vi "PH_SSAC.panel.vi"(0 "object ref":refnum<vi>, 5 "error in (no error)":errorcluster) -> (19 "error out":errorcluster)   [LabVIEW 2014, in "PH_SSAC.lvlib"]
doc: "This a GUI.\n\nLicense Agreement for this software:\n\nCopyright (C)\nGesellschaft für Schwerionenforschung, GSI\nPlanckstr. 1\n64291 Darmstadt\nGermany\n\nContact: D.Beck@gsi.de \n\nThis program is free software; you can redistribute it and/or modify it under the terms of the GNU General Public License as published by the Free Software Foundation; either version 2 of the license, or (at your option) any later version.\n\nThis program is distributed in the hope that it will be useful, but WITHOUT ANYW ARRANTY; without even the implied warranty of MERCHANTABILITY or FITNESS FOR A PARTICULAR PURPOSE. See the GNU General License for more details (http://www.gnu.org).\n\nGesellschaft für Schwerionenforschung, GSI\nPlanckstr. 1, 64291 Darmstadt, Germany\nFor all questions and ideas contact: M.Richter@gsi.de, H.Brand@gsi.de or D.Beck@gsi.de.\nLast update: 18-DEC-2002"
uses:
  PH_SSAC.lvlib
  PH_Basics/PH_StatusHandler/PH_StatusHandler.GUI element.ctl
  PH_SSAC.Background Data.ctl
  PH_Basics/PH_Img_BaseClass/PH_Img_BaseClass.Palette.ctl
  PH_Basics/PH_Img_BaseClass/PH_Img_BaseClass.GUI Refs.ctl
  PH_SSAC.Signal Selector.ctl
  PH_Basics/PH_StatusHandler/PH_StatusHandler.Status.ctl
  CS_Core/CSObj/CSObj.lvlib
  PH_Basics/PH_Common/PH_Common.lvlib
  CS_Core/CSSystem/CSSystemLib/CSSystemLib.lvlib
  PH_Basics/PH_Img_BaseClass/PH_Img_BaseClass.lvlib
  PH_Basics/PH_Class/PH_Class.lvlib
  PH_Basics/PH_PSDBWriter/PH_PSDBWriter.lvlib
  PH_Basics/PH_StatusHandler/PH_StatusHandler.lvlib
panel:
  out "Background":u32(colorbox)=16860
  out "Timeout":u32(colorbox)=16860
  in  "Tab Control":T1(tab)=enum."Calibration"
  in  "Export Evaluation":bool caption="Export\nEvaluation"
  in  "# for Average":i32=1
  out "Saturation":bool
  out "Processed":bool
  in  "Threshold":dbl
  out "Mean Pulse Duration":dbl caption="fs"
  out "Current Pulse Duration":dbl caption="fs"
  out "Time evolution of mean pulse duration":dbl[](graph)
  out "Main signal":cluster{dbl[], "Main Signal":dbl[]}(graph)
  out "Calibration Factor":dbl caption="fs/pixel"
  in  "dt":dbl=1.0 caption="fs"
  out "Cam Source":string
  in  "Timeout Set":i32 caption="ms"
  in  "Global On":bool caption="On"
  in  "Palette":T2 items=["Grey", "Binary", "Gradient", "Rainbow", "Temperature"]
  out "GUI Image":T3(plugin-control)
  in  "Frame Main":cluster{"x":u32, "dx":u32, "y":u32, "dy":u32}={"x"=0, "dx"=1280, "y"=150, "dy"=150} caption="Main Signal"
  in  "Frame Background":cluster{"x":u32, "dx":u32, "y":u32, "dy":u32}={"x"=0, "dx"=100, "y"=400, "dy"=250} caption="Background"
  in  "Calibration Procedure":bool
  out "Background Calibration Data":T4={"Date"="", "Time"="", "Frame Main"={"x"=0, "dx"=0, "y"=0, "dy"=0}, "dt [fs]"=0.0, "Calibration Factor [fs/pixel]"=0.0, "Signal"=array[1280 elements], "Frame Background"={"x"=0, "dx"=100, "y"=400, "dy"=250}}
  in  "Read BG Data":bool
  in  "Save BG Data":bool
  out "Current Position":i32 caption="pixel"
  in  "Background acquire":bool
  out "Resulting Factor":dbl caption="fs/pixel"
  in  "Stage Pos 1":dbl caption="mm"
  in  "1st peak at":dbl caption="pixel"
  in  "2nd peak at":dbl caption="pixel"
  in  "Stage Pos 2":dbl caption="mm"
  in  "Calculate Factor":bool
  in  "Calibration Procedure Step":u16(ring)
  out "PSDB Status":u32(colorbox)=6618880 caption="PSDB"
  out "Status":T5 caption="Enabling State"
  in  "Delete":bool
  in  "Exit":bool
  # "PCS"
  # "3.40"
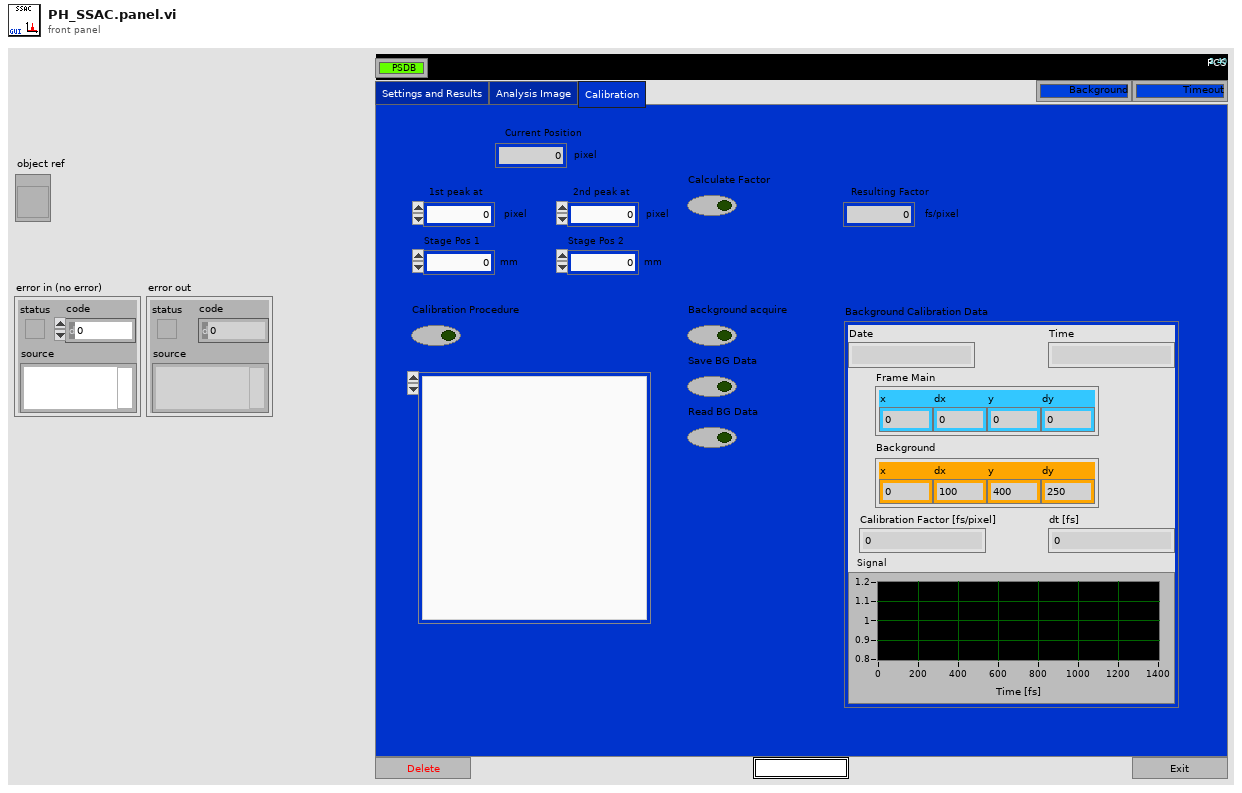
[diagram p1: front panel]
types:
  T1 = enum32{"Settings and Results", "Analysis Image", "Calibration"}
  T2 = typedef "PH_Img_BaseClass.lvlib/PH_Img_BaseClass.Palette.ctl" = i32
  T3 = typedef "IMAQ Image.ctl" = refnum<image>
  T4 = typedef "PH_SSAC.lvlib/PH_SSAC.Background Data.ctl" = cluster{"Date":string, "Time":string, "Frame Main":cluster{"x":u32, "dx":u32, "y":u32, "dy":u32}, "dt [fs]":dbl, "Calibration Factor [fs/pixel]":dbl, "Signal":dbl[], "Frame Background":cluster{"x":u32, "dx":u32, "y":u32, "dy":u32}}
  T5 = typedef "PH_StatusHandler.lvlib/PH_StatusHandler.GUI element.ctl" = u16
  T6 = typedef "PH_Img_BaseClass.lvlib/PH_Img_BaseClass.GUI Refs.ctl" = cluster{"Timeout":refnum<vi>, "Image":refnum<vi>, "Palette":refnum<vi>, "Timeout Set":refnum<vi>}
  T7 = typedef "PH_SSAC.lvlib/PH_SSAC.Signal Selector.ctl" = enum16{"Main", "Background"}
  T8 = typedef "PH_SSAC.lvlib/PH_SSAC.i attribute.ctl" = cluster{"GUI Refs":cluster{"Delete":refnum<vi>, "Global On":refnum<vi>, "Cam Source":refnum<vi>, "Frame Main Signal":refnum<vi>, "Frame Background":refnum<vi>, "dt (Gauss smooth)":refnum<vi>, "Calibration Factor":refnum<vi>, "Background acquire":refnum<vi>, "Threshold":refnum<vi>, "Time evolution of mean pulse duration":refnum<vi>, "Mean Pulse Duration":refnum<vi>, "Main signal":refnum<vi>, "Current Pulse Duration":refnum<vi>, "Processed":refnum<vi>, "Saturation":refnum<vi>, "# for Average":refnum<vi>, "Position":refnum<vi>, "BG Status":refnum<vi>, "Save BG data":refnum<vi>, "Read BG Data":refnum<vi>, "Background Calibration Data":refnum<vi>}, "Images":cluster{"OP Image":T3, "GUI Image":T3, "PSDB Image":T3}, "Global On?":bool, "Frame Main":cluster{"x":u32, "dx":u32, "y":u32, "dy":u32}, "Frame Background":cluster{"x":u32, "dx":u32, "y":u32, "dy":u32}, "dt [fs]":dbl, "Calibration Factor [fs/pixel]":dbl, "Threshold":dbl, "Time evolution of mean pulse duration [fs]":dbl[], "Main Signal":cluster{"Time for Main":dbl[], "Signal":dbl[]}, "Processed":bool, "Current Pulse Duration [fs]":dbl, "# for Average":i32, "Position":i32, "Pulse Durations [fs]":dbl[], "BG":cluster{"Acquire?":bool, "Background Calibration Data":T4, "Save Data":bool}}
  T9 = typedef "PH_StatusHandler.lvlib/PH_StatusHandler.Status.ctl" = i16
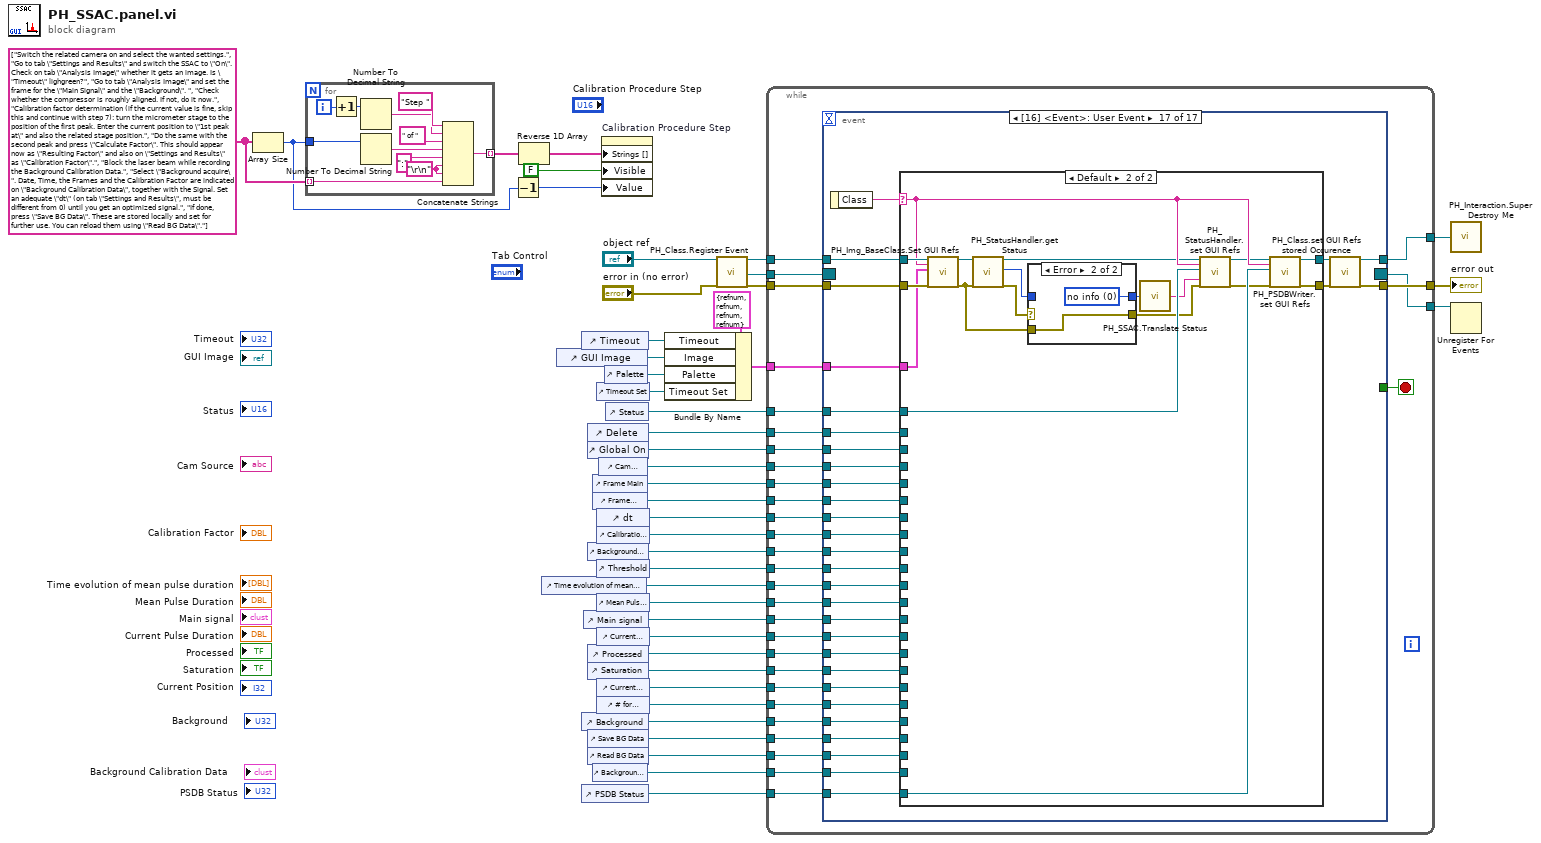
[diagram p0: block diagram]
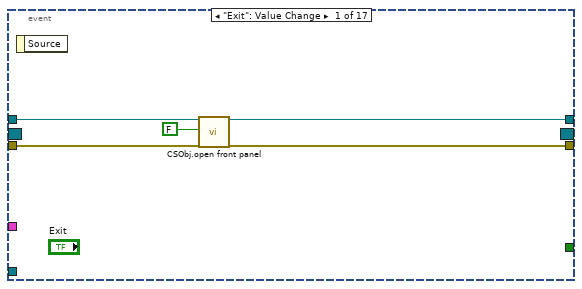
[diagram p2: hidden frame]
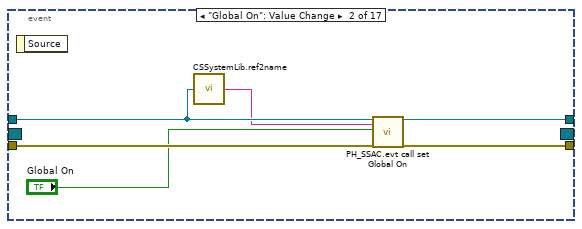
[diagram p3: hidden frame]
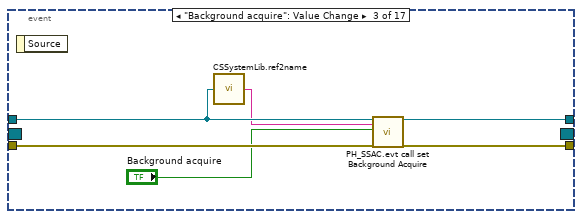
[diagram p4: hidden frame]
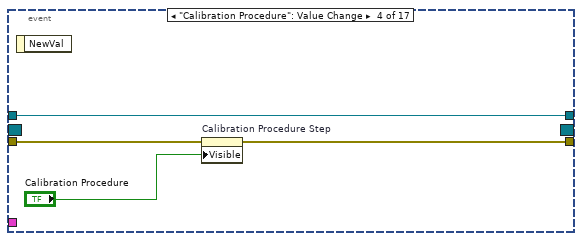
[diagram p5: hidden frame]
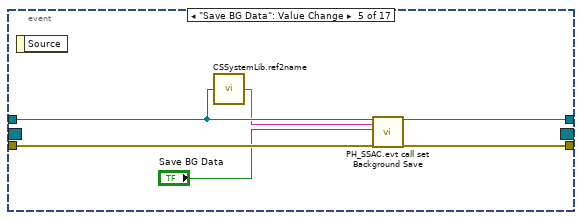
[diagram p6: hidden frame]
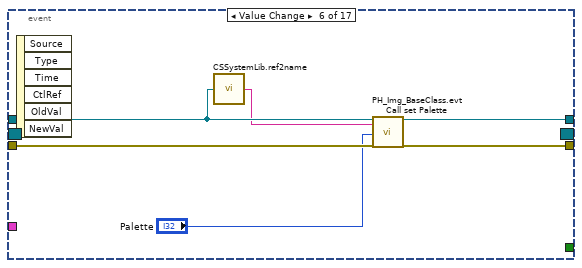
[diagram p7: hidden frame]
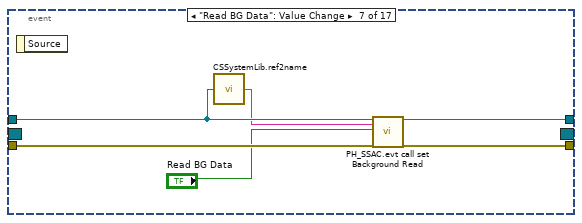
[diagram p8: hidden frame]
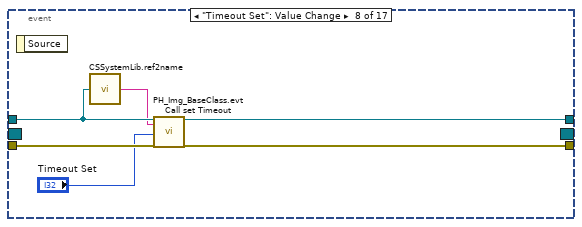
[diagram p9: hidden frame]
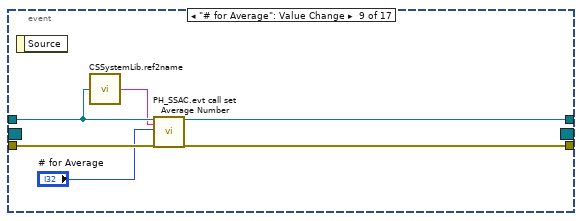
[diagram p10: hidden frame]
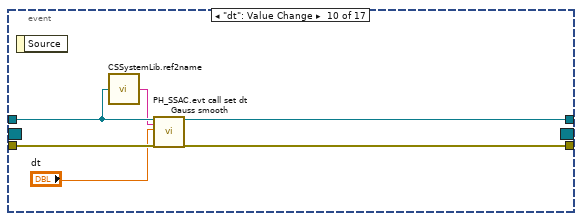
[diagram p11: hidden frame]
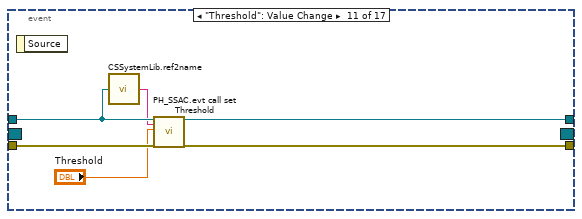
[diagram p12: hidden frame]
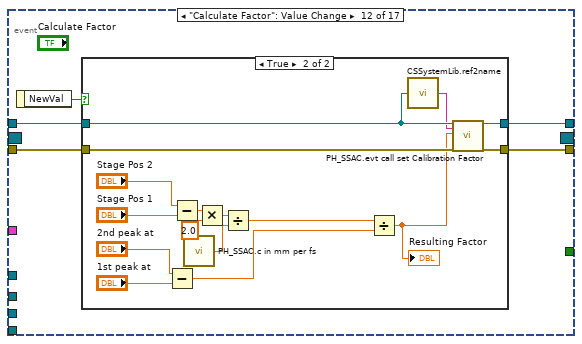
[diagram p13: hidden frame]
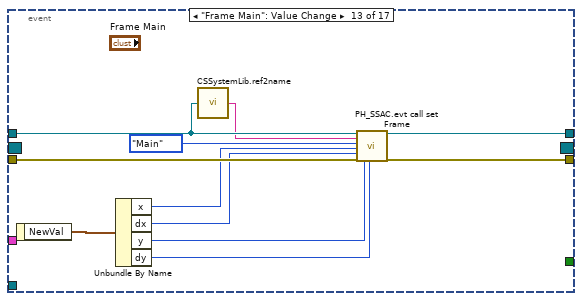
[diagram p15: hidden frame]
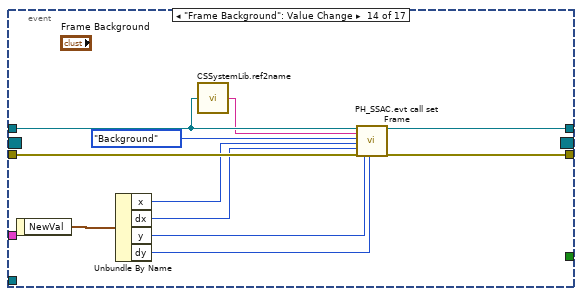
[diagram p16: hidden frame]
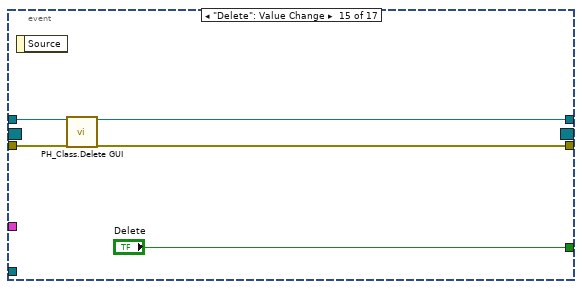
[diagram p17: hidden frame]
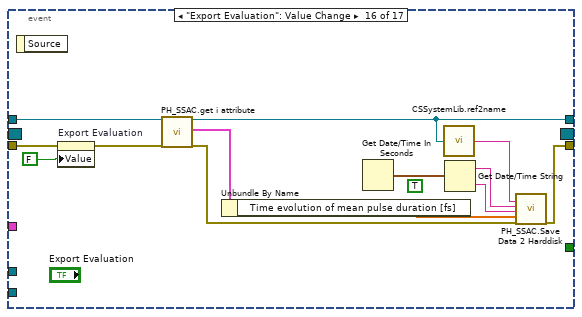
[diagram p18: hidden frame]
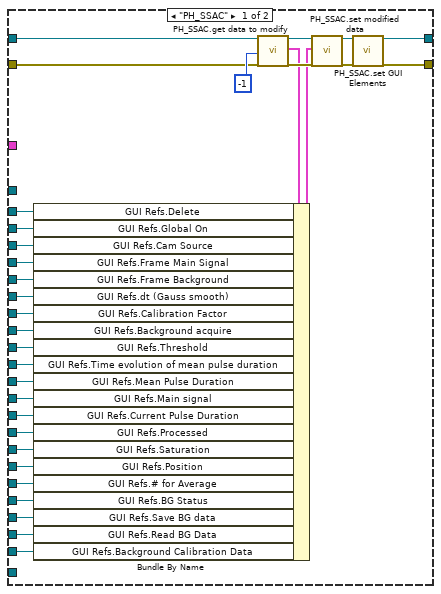
[diagram p19: hidden frame]
diagram:
  w40 = string[] ["Switch the related camera on and select the wanted settings.", "Go to tab \"Settings and Results\" and switch the SSAC to \"On\". Check on tab \"Analysis Image\" whether it gets an image. Is \"Timeout\" lighgreen?", "Go to tab \"Analysis Image\" and set the frame for the \"Main Signal\" and the \"Background\". ", "Check whether the compressor is roughly aligned. If not, do it now.", "Calibration factor determination (if the current value is fine, skip this and continue with step 7): turn the micrometer stage to the position of the first peak. Enter the current position to \"1st peak at\" and also the related stage position.", "Do the same with the second peak and press \"Calculate Factor\". This should appear now as \"Resulting Factor\" and also on \"Settings and Results\" as \"Calibration Factor\".", "Block the laser beam while recording the Background Calibration Data.", "Select \"Background acquire\". Date, Time, the Frames and the Calibration Factor are indicated on \"Background Calibration Data\", together with the Signal. Set an adequate \"dt\" (on tab \"Settings and Results\", must be different from 0) until you get an optimized signal.", "If done, press \"Save BG Data\". These are stored locally and set for further use. You can reload them using \"Read BG Data\"."]
  n1 = Array Size(array=w40) -> (size(s)=w36:i32)
  n2 = for {
    tunnel: w40 -> [w44] mode=indexing
    tunnel: [w53] -> w38 mode=indexing
    tunnel: w36 -> [w48]
    i -> [w52]
    w45 = "\r\n"
    n3 = Increment(x=w52) -> (x+1=w51:i32)
    n4 = Number To Decimal String(number=w51) -> (decimal integer string=w50:string)  [unwired: 1 in]
    n5 = Number To Decimal String(number=w48) -> (decimal integer string=w47:string)  [unwired: 1 in]
    n6 = Concatenate Strings("Step " ("string"), w50, " of " ("string"), w47, ":" ("string"), w45, w45, w44) -> (w53:string)
  }
  n7 = Decrement(x=w36) -> (x-1=w37:i32)
  n8 = Reverse 1D Array(array=w38) -> (reversed array=w39:string[])
  n9 = control-ref of="Time evolution of mean pulse duration"() -> (w16:refnum<vi>)
  n10 = control-ref of="GUI Image"() -> (w33:refnum<vi>)
  n11 = control-ref of="Timeout"() -> (w34:refnum<vi>)
  n12 = control-ref of="Background"() -> (w8:refnum<vi>)
  n13 = control-ref of="PSDB Status"() -> (w26:refnum<vi>)
  n14 = control-ref of="Main signal"() -> (w14:refnum<vi>)
  n15 = control-ref of="Delete"() -> (w25:refnum<vi>)
  n16 = control-ref of="Global On"() -> (w24:refnum<vi>)
  n17 = control-ref of="Background acquire"() -> (w18:refnum<vi>)
  n18 = control-ref of="Processed"() -> (w12:refnum<vi>)
  n19 = control-ref of="Saturation"() -> (w11:refnum<vi>)
  n20 = control-ref of="Save BG Data"() -> (w7:refnum<vi>)
  n21 = control-ref of="Read BG Data"() -> (w6:refnum<vi>)
  n22 = control-ref of="Frame Main"() -> (w22:refnum<vi>)
  n23 = control-ref of="Frame Background"() -> (w21:refnum<vi>)
  n24 = control-ref of="Background Calibration Data"() -> (w5:refnum<vi>)
  n25 = control-ref of="Timeout Set"() -> (w31:refnum<vi>)
  n26 = control-ref of="dt"() -> (w20:refnum<vi>)
  n27 = control-ref of="Calibration Factor"() -> (w19:refnum<vi>)
  n28 = control-ref of="Threshold"() -> (w17:refnum<vi>)
  n29 = control-ref of="Mean Pulse Duration"() -> (w15:refnum<vi>)
  n30 = control-ref of="Current Pulse Duration"() -> (w13:refnum<vi>)
  n31 = control-ref of="Current Position"() -> (w10:refnum<vi>)
  n32 = control-ref of="# for Average"() -> (w9:refnum<vi>)
  n33 = control-ref of="Cam Source"() -> (w23:refnum<vi>)
  n34 = property on="Calibration Procedure Step" class="Ring (strict)"("Strings []"=w39, "Visible"=FALSE, "Value"=w37) -> ()  [unwired: 2 in, 2 out]
  n35 = control-ref of="Palette"() -> (w32:refnum<vi>)
  n36 = control-ref of="Status"() -> (w1:refnum<vi>)
  n37 = Bundle By Name(cluster=T6 {"Timeout"=refnum, "Image"=refnum, "Palette"=refnum, "Timeout Set"=refnum} ("GUI Refs"), "Timeout"=w34, "Image"=w33, "Palette"=w32, "Timeout Set"=w31) -> (w4:T6)
  n38 = call "PH_Class.Register Event.vi"("i ref in"="object ref", "error in (no error)"="error in (no error)") -> ("i ref out"=w29:refnum<vi>, "Event Registration Refnum"=w28:refnum<event-registration>, "error out"=w30:errorcluster)  [unwired: 15 in]
  n39 = while {
    tunnel: w29 -> [w82]
    tunnel: [w81] -> w43
    tunnel: w30 -> [w84]
    tunnel: [w83] -> w42
    tunnel: w28 -> [w80]
    tunnel: [w79] -> w27
    tunnel: w26 -> [w78]
    tunnel: w25 -> [w77]
    tunnel: w1 -> [w76]
    tunnel: w24 -> [w75]
    tunnel: w23 -> [w74]
    tunnel: w22 -> [w73]
    tunnel: w21 -> [w72]
    tunnel: w20 -> [w71]
    tunnel: w19 -> [w70]
    tunnel: w18 -> [w69]
    tunnel: w17 -> [w68]
    tunnel: w16 -> [w67]
    tunnel: w15 -> [w66]
    tunnel: w14 -> [w65]
    tunnel: w13 -> [w64]
    tunnel: w12 -> [w63]
    tunnel: w11 -> [w62]
    tunnel: w10 -> [w61]
    tunnel: w9 -> [w60]
    tunnel: w8 -> [w59]
    tunnel: w7 -> [w58]
    tunnel: w6 -> [w57]
    tunnel: w5 -> [w56]
    tunnel: w4 -> [w55]
    stop <- w85 stop-if-true
    n40 = event shown="[16] <Event>: User Event" {
      selector: w80 -> [_ _ _ _ _ _ _ _ _ _ _ _ _ _ _ _ _]
      dyn-events: [_ _ _ _ _ _ _ _ _ _ _ _ _ _ _ _ _] -> w79
      timeout: _ -> [_ _ _ _ _ _ _ _ _ _ _ _ _ _ _ _ _]
      tunnel: [_ _ _ _ _ _ _ _ _ _ _ _ _ _ "Delete" _ _] -> w85
      tunnel: w82 -> [w87 w92 w99 w103 w109 w115 w121 w127 w133 w139 w145 w150 w179 w190 w197 w209 w242]
      tunnel: w84 -> [w90 w96 w102 w106 w112 w118 w124 w130 w136 w142 w148 w153 w182 w193 w196 w210 w239]
      tunnel: [w89 w95 w101 w105 w111 w117 w123 w129 w135 w141 w147 w152 w181 w192 w194 w204 w237] -> w83
      tunnel: [w86 w94 w100 w103 w110 w116 w122 w128 w134 w140 w146 w151 w180 w191 w195 w199 w240] -> w81
      tunnel: w78 -> [_ _ _ _ _ _ _ _ _ _ _ _ _ _ _ _ w236]
      tunnel: w77 -> [_ _ _ _ _ _ _ _ _ _ _ _ _ _ _ _ w234]
      tunnel: w76 -> [_ _ _ _ _ _ _ _ _ _ _ _ _ _ _ _ w233]
      tunnel: w75 -> [_ _ _ _ _ _ _ _ _ _ _ _ _ _ _ _ w232]
      tunnel: w74 -> [_ _ _ _ _ _ _ _ _ _ _ _ _ _ _ _ w231]
      tunnel: w73 -> [_ _ _ _ _ _ _ _ _ _ _ _ _ _ _ _ w230]
      tunnel: w72 -> [_ _ _ _ _ _ _ _ _ _ _ _ _ _ _ _ w229]
      tunnel: w71 -> [_ _ _ _ _ _ _ _ _ _ _ _ _ _ _ _ w228]
      tunnel: w70 -> [_ _ _ _ _ _ _ _ _ _ _ _ _ _ _ _ w227]
      tunnel: w69 -> [_ _ _ _ _ _ _ _ _ _ _ _ _ _ _ _ w226]
      tunnel: w68 -> [_ _ _ _ _ _ _ _ _ _ _ _ _ _ _ _ w225]
      tunnel: w67 -> [_ _ _ _ _ _ _ _ _ _ _ _ _ _ _ _ w224]
      tunnel: w66 -> [_ _ _ _ _ _ _ _ _ _ _ _ _ _ _ _ w223]
      tunnel: w65 -> [_ _ _ _ _ _ _ _ _ _ _ _ _ _ _ _ w222]
      tunnel: w64 -> [_ _ _ _ _ _ _ _ _ _ _ _ _ _ _ _ w221]
      tunnel: w63 -> [_ _ _ _ _ _ _ _ _ _ _ _ _ _ _ _ w220]
      tunnel: w62 -> [_ _ _ _ _ _ _ _ _ _ _ _ _ _ _ _ w219]
      tunnel: w61 -> [_ _ _ _ _ _ _ _ _ _ _ _ _ _ _ _ w218]
      tunnel: w60 -> [_ _ _ _ _ _ _ _ _ _ _ _ _ _ _ _ w217]
      tunnel: w59 -> [_ _ _ _ _ _ _ _ _ _ _ _ _ _ _ _ w216]
      tunnel: w58 -> [_ _ _ _ _ _ _ _ _ _ _ _ _ _ _ _ w215]
      tunnel: w57 -> [_ _ _ _ _ _ _ _ _ _ _ _ _ _ _ _ w214]
      tunnel: w56 -> [_ _ _ _ _ _ _ _ _ _ _ _ _ _ _ _ w213]
      tunnel: w55 -> [_ _ _ _ _ _ _ _ _ _ _ _ _ _ _ _ w212]
      event "Exit": Value Change {
        n41 = event-data() -> ()  [unwired: 1 in, 1 out]
        n42 = call "CSObj.open front panel.vi"("i ref in"=w87, "frontPanelOpen"=FALSE ("front panel open"), "error in (no error)"=w90) -> ("i ref out"=w86:refnum<vi>, "error out"=w89:errorcluster)  [unwired: 15 in]
      }
      event "Global On": Value Change {
        n43 = event-data() -> ()  [unwired: 1 in, 1 out]
        n44 = call "CSSystemLib.ref2name.vi"("obj refnum"=w92) -> ("name"=w91:string)
        n45 = call "PH_SSAC.evt call set Global On.vi"("i ref in"=w92, "Instance"=w91, "Global On"="Global On", "error in (no error)"=w96) -> ("i ref out"=w94:refnum<vi>, "error out"=w95:errorcluster)  [unwired: 14 in]
      }
      event "Background acquire": Value Change {
        n46 = event-data() -> ()  [unwired: 1 in, 1 out]
        n47 = call "CSSystemLib.ref2name.vi"("obj refnum"=w99) -> ("name"=w98:string)
        n48 = call "PH_SSAC.evt call set Background Acquire.vi"("i ref in"=w99, "Instance"=w98, "Background Acquire"="Background acquire", "error in (no error)"=w102) -> ("i ref out"=w100:refnum<vi>, "error out"=w101:errorcluster)  [unwired: 14 in]
      }
      event "Calibration Procedure": Value Change {
        n49 = event-data() -> ()  [unwired: 1 in, 1 out]
        n50 = property on="Calibration Procedure Step" class="Ring (strict)"(error in=w106, "Visible"="Calibration Procedure") -> (error out=w105:errorcluster)  [unwired: 1 in, 1 out]
      }
      event "Save BG Data": Value Change {
        n51 = event-data() -> ()  [unwired: 1 in, 1 out]
        n52 = call "CSSystemLib.ref2name.vi"("obj refnum"=w109) -> ("name"=w108:string)
        n53 = call "PH_SSAC.evt call set Background Save.vi"("i ref in"=w109, "Instance"=w108, "Background Save"="Save BG Data", "error in (no error)"=w112) -> ("i ref out"=w110:refnum<vi>, "error out"=w111:errorcluster)  [unwired: 14 in]
      }
      event Value Change {
        n54 = event-data() -> ()  [unwired: 1 in, 6 out]
        n55 = call "CSSystemLib.ref2name.vi"("obj refnum"=w115) -> ("name"=w114:string)
        n56 = call "PH_Img_BaseClass.evt Call set Palette.vi"("i ref in"=w115, "Instance"=w114, "Palette"="Palette", "error in (no error)"=w118) -> ("i ref out"=w116:refnum<vi>, "error out"=w117:errorcluster)  [unwired: 14 in]
      }
      event "Read BG Data": Value Change {
        n57 = event-data() -> ()  [unwired: 1 in, 1 out]
        n58 = call "CSSystemLib.ref2name.vi"("obj refnum"=w121) -> ("name"=w120:string)
        n59 = call "PH_SSAC.evt call set Background Read.vi"("i ref in"=w121, "Instance"=w120, "Background Read"="Read BG Data", "error in (no error)"=w124) -> ("i ref out"=w122:refnum<vi>, "error out"=w123:errorcluster)  [unwired: 14 in]
      }
      event "Timeout Set": Value Change {
        n60 = event-data() -> ()  [unwired: 1 in, 1 out]
        n61 = call "CSSystemLib.ref2name.vi"("obj refnum"=w127) -> ("name"=w126:string)
        n62 = call "PH_Img_BaseClass.evt Call set Timeout.vi"("i ref in"=w127, "Instance"=w126, "Timeout [ms]"="Timeout Set", "error in (no error)"=w130) -> ("i ref out"=w128:refnum<vi>, "error out"=w129:errorcluster)  [unwired: 14 in]
      }
      event "# for Average": Value Change {
        n63 = event-data() -> ()  [unwired: 1 in, 1 out]
        n64 = call "CSSystemLib.ref2name.vi"("obj refnum"=w133) -> ("name"=w132:string)
        n65 = call "PH_SSAC.evt call set Average Number.vi"("i ref in"=w133, "Instance"=w132, "Timeout Set"="# for Average", "error in"=w136) -> ("i ref out"=w134:refnum<vi>, "error out"=w135:errorcluster)  [unwired: 14 in]
      }
      event "dt": Value Change {
        n66 = event-data() -> ()  [unwired: 1 in, 1 out]
        n67 = call "CSSystemLib.ref2name.vi"("obj refnum"=w139) -> ("name"=w138:string)
        n68 = call "PH_SSAC.evt call set dt Gauss smooth.vi"("i ref in"=w139, "Instance"=w138, "dt (Gauss smooth)"="dt", "error in"=w142) -> ("i ref out"=w140:refnum<vi>, "error out"=w141:errorcluster)  [unwired: 14 in]
      }
      event "Threshold": Value Change {
        n69 = event-data() -> ()  [unwired: 1 in, 1 out]
        n70 = call "CSSystemLib.ref2name.vi"("obj refnum"=w145) -> ("name"=w144:string)
        n71 = call "PH_SSAC.evt call set Threshold.vi"("i ref in"=w145, "Instance"=w144, "Threshold"="Threshold", "error in"=w148) -> ("i ref out"=w146:refnum<vi>, "error out"=w147:errorcluster)  [unwired: 14 in]
      }
      event "Calculate Factor": Value Change {
        n72 = event-data() -> ("NewVal"=w149:bool)  [unwired: 1 in]
        n73 = case shown="True" w149 {
          tunnel: w153 -> [w154 w171]
          tunnel: [w154 w170] -> w152
          tunnel: [w155 w169] -> w151
          tunnel: w150 -> [w155 w168]
          frame False {
          }
          frame True {
            n74 = Subtract(x="2nd peak at", y="1st peak at") -> (x-y=w158:dbl)
            n75 = Subtract(x="Stage Pos 2", y="Stage Pos 1") -> (x-y=w166:dbl)
            n76 = call "PH_SSAC.c in mm per fs.vi"() -> ("c [mm/fs]"=w156:dbl)
            n77 = Multiply(x=w166, y=2.0) -> (x*y=w165:dbl)
            n78 = Divide(x=w165, y=w156) -> (x/y=w164:dbl)
            n79 = Divide(x=w164, y=w158) -> (x/y=w157:dbl)
            "Resulting Factor" <- w157
            n80 = call "CSSystemLib.ref2name.vi"("obj refnum"=w168) -> ("name"=w167:string)
            n81 = call "PH_SSAC.evt call set Calibration Factor.vi"("i ref in"=w168, "Instance"=w167, "calibration Factor [fs/pixel]"=w157, "error in"=w171) -> ("i ref out"=w169:refnum<vi>, "error out"=w170:errorcluster)  [unwired: 14 in]
          }
        }
      }
      event "Frame Main": Value Change {
        n82 = event-data() -> ("NewVal"=w177:cluster{"x":u32, "dx":u32, "y":u32, "dy":u32})  [unwired: 1 in]
        n83 = Unbundle By Name(w177) -> ("x"=w176:u32, "dx"=w175:u32, "y"=w174:u32, "dy"=w173:u32)
        n84 = call "CSSystemLib.ref2name.vi"("obj refnum"=w179) -> ("name"=w178:string)
        n85 = call "PH_SSAC.evt call set Frame.vi"("i ref in"=w179, "Instance"=w178, "Signal"=PH_SSAC.Signal_Selector."Main", "x"=w176, "dx"=w175, "error in"=w182, "y"=w174, "dy"=w173) -> ("i ref out"=w180:refnum<vi>, "error out"=w181:errorcluster)  [unwired: 10 in]
      }
      event "Frame Background": Value Change {
        n86 = event-data() -> ("NewVal"=w188:cluster{"x":u32, "dx":u32, "y":u32, "dy":u32})  [unwired: 1 in]
        n87 = Unbundle By Name(w188) -> ("x"=w187:u32, "dx"=w186:u32, "y"=w185:u32, "dy"=w184:u32)
        n88 = call "CSSystemLib.ref2name.vi"("obj refnum"=w190) -> ("name"=w189:string)
        n89 = call "PH_SSAC.evt call set Frame.vi"("i ref in"=w190, "Instance"=w189, "Signal"=PH_SSAC.Signal_Selector."Background", "x"=w187, "dx"=w186, "error in"=w193, "y"=w185, "dy"=w184) -> ("i ref out"=w191:refnum<vi>, "error out"=w192:errorcluster)  [unwired: 10 in]
      }
      event "Delete": Value Change {
        n90 = event-data() -> ()  [unwired: 1 in, 1 out]
        n91 = call "PH_Class.Delete GUI.vi"("VI in"=w197, "error in (no error)"=w196) -> ("VI out"=w195:refnum<vi>, "error out"=w194:errorcluster)  [unwired: 16 in]
      }
      event "Export Evaluation": Value Change {
        (unwired) TRUE ("want seconds? (F)")
        n92 = event-data() -> ()  [unwired: 1 in, 1 out]
        n93 = property on="Export Evaluation" class="Bool (strict)"(error in=w210, "Value"=FALSE ("Export Evaluation")) -> (error out=w208:errorcluster)  [unwired: 1 in, 1 out]
        n94 = call "PH_SSAC.get i attribute.vi"("i ref in"=w209, "error in (no error)"=w208) -> ("i ref out"=w199:refnum<vi>, "i attribute"=w207:T8, "error out"=w205:errorcluster)  [unwired: 15 in]
        n95 = Unbundle By Name(w207) -> ("Time evolution of mean pulse duration [fs]"=w206:dbl[])
        n96 = Get Date/Time In Seconds() -> (seconds since 1Jan1904=w203:timestamp)
        n97 = call "CSSystemLib.ref2name.vi"("obj refnum"=w199) -> ("name"=w200:string)
        n98 = Get Date/Time String(seconds (now)=w203) -> (date string=w201:string, time string=w202:string)  [unwired: 2 in]
        n99 = call "PH_SSAC.Save Data 2 Harddisk.vi"("Instance Name"=w200, "Date"=w201, "Time"=w202, "Time evolution of mean pulse duration [fs]"=w206, "error in"=w205) -> ("error out"=w204:errorcluster)  [unwired: 14 in]
      }
      event User Event {
        n100 = event-data() -> ("Class"=w235:string)  [unwired: 1 in]
        n101 = case shown="Default" w235 {
          selector: w235 -> [_ w285]
          tunnel: w242 -> [w271 w292]
          tunnel: [w245 w288] -> w241
          tunnel: w239 -> [w270 w291]
          tunnel: [w243 w289] -> w238
          tunnel: w236 -> [_ w287]
          tunnel: w234 -> [w267 _]
          tunnel: w233 -> [_ w284]
          tunnel: w232 -> [w266 _]
          tunnel: w231 -> [w265 _]
          tunnel: w230 -> [w264 _]
          tunnel: w229 -> [w263 _]
          tunnel: w228 -> [w262 _]
          tunnel: w227 -> [w261 _]
          tunnel: w226 -> [w260 _]
          tunnel: w225 -> [w259 _]
          tunnel: w224 -> [w258 _]
          tunnel: w223 -> [w257 _]
          tunnel: w222 -> [w256 _]
          tunnel: w221 -> [w255 _]
          tunnel: w220 -> [w254 _]
          tunnel: w219 -> [w253 _]
          tunnel: w218 -> [w252 _]
          tunnel: w217 -> [w251 _]
          tunnel: w216 -> [w250 _]
          tunnel: w215 -> [w249 _]
          tunnel: w214 -> [w248 _]
          tunnel: w213 -> [w247 _]
          tunnel: w212 -> [_ w290]
          frame "PH_SSAC" {
            n102 = call "PH_SSAC.get data to modify.vi"("i ref in"=w271, "ms timeout (10000)"=-1, "error in (no error)"=w270) -> ("i ref out"=w274:refnum<vi>, "i attribute"=w269:T8, "error out"=w273:errorcluster)  [unwired: 13 in, 1 out]
            n103 = Bundle By Name(cluster=w269, "GUI Refs.Delete"=w267, "GUI Refs.Global On"=w266, "GUI Refs.Cam Source"=w265, "GUI Refs.Frame Main Signal"=w264, "GUI Refs.Frame Background"=w263, "GUI Refs.dt (Gauss smooth)"=w262, "GUI Refs.Calibration Factor"=w261, "GUI Refs.Background acquire"=w260, "GUI Refs.Threshold"=w259, "GUI Refs.Time evolution of mean pulse duration"=w258, "GUI Refs.Mean Pulse Duration"=w257, "GUI Refs.Main signal"=w256, "GUI Refs.Current Pulse Duration"=w255, "GUI Refs.Processed"=w254, "GUI Refs.Saturation"=w253, "GUI Refs.Position"=w252, "GUI Refs.# for Average"=w251, "GUI Refs.BG Status"=w250, "GUI Refs.Save BG data"=w249, "GUI Refs.Read BG Data"=w248, "GUI Refs.Background Calibration Data"=w247) -> (w268:T8)
            n104 = call "PH_SSAC.set modified data.vi"("i ref in"=w274, "i attribute"=w268, "error in (no error)"=w273) -> ("i ref out"=w246:refnum<vi>, "error out"=w244:errorcluster)  [unwired: 15 in]
            n105 = call "PH_SSAC.set GUI Elements.vi"("i ref in"=w246, "error in"=w244) -> ("i ref out"=w245:refnum<vi>, "error out"=w243:errorcluster)  [unwired: 16 in]
          }
          frame Default {
            n106 = call "PH_Img_BaseClass.Set GUI Refs.vi"("i ref in"=w292, "Class"=w285, "GUI Refs"=w290, "error in (no error)"=w291) -> ("i ref out"=w282:refnum<vi>, "error out"=w275:errorcluster)  [unwired: 14 in]
            n107 = call "PH_StatusHandler.get Status.vi"("VI in"=w282, "error in"=w275) -> ("VI out"=w281:refnum<vi>, "Status"=w279:T9, "error out"=w280:errorcluster)  [unwired: 15 in]
            n108 = case shown="Error" w280 {
              selector: w280 -> [w293 _]
              tunnel: w279 -> [w294 _]
              tunnel: [w294 w296] -> w278
              tunnel: [w293 w295] -> w276
              tunnel: w275 -> [_ w295]
              frame No Error {
              }
              frame Error {
                w296 = T9 0 items=["no info", "off/false/out", "on/true/in", "Failure", "Alarm", "Status 1", "Status 2", "Status 3"] ("Status")
              }
            }
            n109 = call "PH_SSAC.Translate Status.vi"("Device Status"=w278) -> ("Translated Status"=w277:string)
            n110 = call "PH_StatusHandler.set GUI Refs.vi"("i ref in"=w281, "Class"=w285, "GUI Ref"=w284, "Tip Strip"=w277, "error in (no error)"=w276) -> ("i ref out"=w283:refnum<vi>, "error out"=w286:errorcluster)  [unwired: 13 in]
            n111 = call "PH_PSDBWriter.set GUI Refs.vi"("i ref in"=w283, "Class"=w285, "Ref PSDB Status"=w287, "error in"=w286) -> ("i ref out"=w288:refnum<vi>, "error out"=w289:errorcluster)  [unwired: 14 in]
          }
        }
        n112 = call "PH_Class.set GUI Refs stored Occurence.vi"("i ref in"=w241, "error in (no error)"=w238) -> ("i ref out"=w240:refnum<vi>, "error out"=w237:errorcluster)  [unwired: 16 in]
      }
    }
  }
  "error out" <- w42
  n113 = call "PH_Interaction.Super Destroy Me.vi"("i ref out"=w43) -> ()
  n114 = Unregister For Events(event registration refnum=w27) -> ()  [unwired: 1 in, 1 out]
